vi "Read Command.vi"(8 "error in (no error)":errorcluster, 11 "Arduino in":refnum<class "Arduino.lvclass">) -> (0 "error out":errorcluster, 2 "read buffer":string, 3 "Arduino out":refnum<class "Arduino.lvclass">)   [LabVIEW 2020, in "Arduino.lvclass"]
doc: "Read command es un vi generico para leer todo lo que el microcontrolador responde despues de hacer cualquier acción"
uses:
  Arduino.lvclass
  Arduino.lvclass/Arduino.ctl
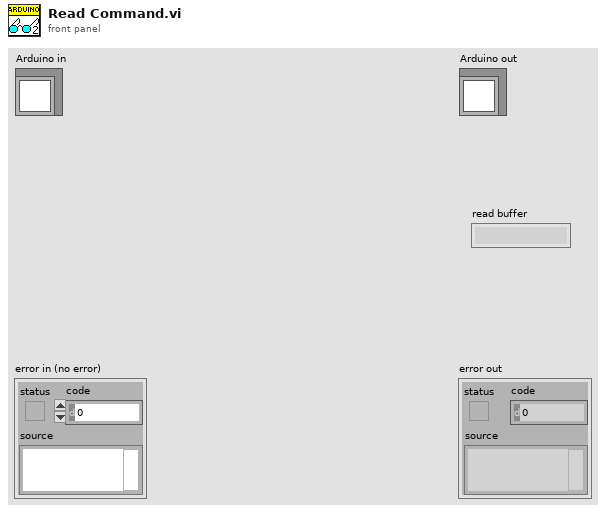
[diagram p1: front panel]
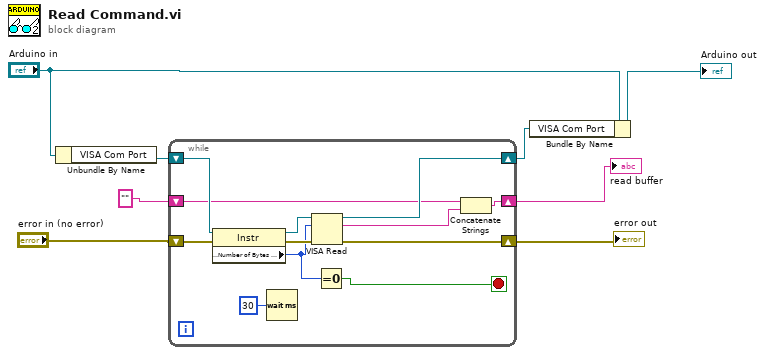
[diagram p0: block diagram]
diagram:
  n1 = Unbundle By Name("Arduino in") -> ("VISA Com Port"=w7:refnum<visa-resource-name>)
  n2 = while {
    shift-right: [w20] -> w2
    shift-left: "error in (no error)" -> [w15]
    shift-right: [w19] -> w8
    shift-left: w7 -> [w17]
    shift-right: [w11] -> w3
    shift-left: "" -> [w10]
    stop <- w12 stop-if-true
    n3 = property class="Instr"(reference=w17, error in=w15) -> (reference out=w16:refnum<visa-resource-name>, error out=w14:errorcluster, "Serial Settings:Number of Bytes at Serial Port"=w13:u32)
    n4 = Wait (ms)(milliseconds to wait=u32 30) -> ()  [unwired: 1 out]
    n5 = VISA Read(VISA resource name=w16, byte count=w13, error in (no error)=w14) -> (VISA resource name out=w19:refnum<visa-resource-name>, read buffer=w18:string, error out=w20:errorcluster)  [unwired: 1 out]
    n6 = Equal To 0?(x=w13) -> (x = 0?=w12:bool)
    n7 = Concatenate Strings(w10, w18) -> (w11:string)
  }
  "error out" <- w2
  "read buffer" <- w3
  n8 = Bundle By Name(cluster="Arduino in", "VISA Com Port"=w8) -> (→"Arduino out":refnum<class "Arduino.lvclass">)
